vi "Read Tube Valves.vi"(0 "task in":refnum<k21>, 1 "Error In":errorcluster, 2 "Tube Inlet":bool, 3 "Mix Inlet":bool, 4 "Mix Outlet":bool, 5 "Tube Outlet":bool) -> (14 "task out":refnum<k21>, 15 "Error Out":errorcluster, 16 "Tube Inlet State":bool, 17 "Mix Inlet State":bool, 18 "Mix Outlet State":bool, 19 "Tube Outlet State":bool)   [LabVIEW 2018]
uses:
  <vilib>/DAQmx/write.llb/DAQmx Write (Digital 1D Bool 1Chan 1Samp).vi
  <vilib>/DAQmx/create/channels.llb/DAQmx Create Channel (DO-Digital Output).vi
  <vilib>/DAQmx/miscellaneous.llb/DAQmx Fill In Error Info.vi
panel:
  # "Valve Controls"
  # "TRUE:   valve open\nFALSE:  valve closed"
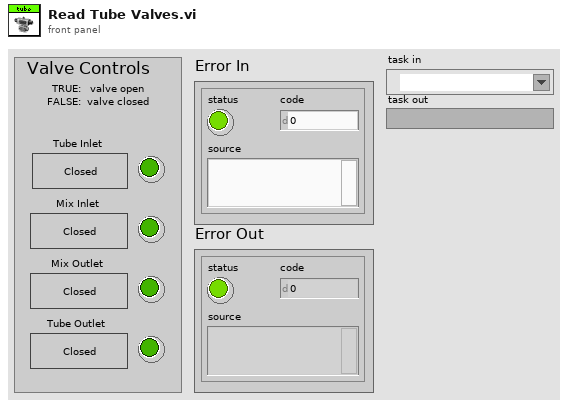
[diagram p1: front panel]
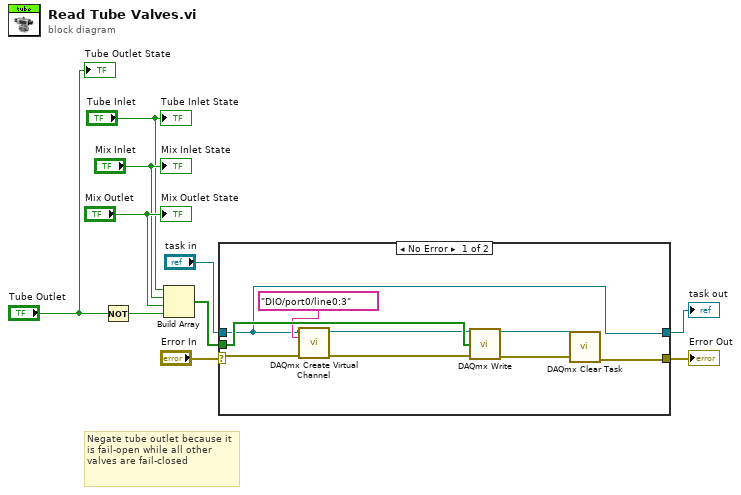
[diagram p0: block diagram]
diagram:
  # "Negate tube outlet because it is fail-open while all other valves are fail-closed"
  n1 = Not(x="Tube Outlet") -> (.not. x?=w8:bool)
  n2 = Build Array("Tube Inlet", "Mix Inlet", "Mix Outlet", w8) -> (w7:bool[])
  n3 = case shown="No Error" "Error In" {
    selector: "Error In" -> [w16 w21]
    tunnel: [w17 w21] -> w9
    tunnel: w7 -> [w19 _]
    tunnel: "task in" -> [w11 w20]
    tunnel: [w11 w20] -> w1
    frame No Error {
      n4 = call-poly <vilib>:"DAQmx Create Virtual Channel.vi"("task in"=w11, "lines"=tag "DIO/port0/line0:3", "error in"=w16) -> ("task out"=w13:refnum<k21>, "error out"=w15:errorcluster)  [unwired: 11 in]
      n5 = call-poly <vilib>:"DAQmx Write.vi"("task/channels in"=w13, "data"=w19, "error in"=w15) -> ("task out"=w12:refnum<k21>, "error out"=w14:errorcluster)  [unwired: 10 in, 1 out]
      n6 = call <vilib>:"DAQmx Clear Task.vi"("task in"=w12, "error in"=w14) -> ("error out"=w17:errorcluster)  [unwired: 13 in]
    }
    frame Error {
    }
  }
  "Error Out" <- w9
  "task out" <- w1
  "Tube Inlet State" <- "Tube Inlet"
  "Mix Inlet State" <- "Mix Inlet"
  "Mix Outlet State" <- "Mix Outlet"
  "Tube Outlet State" <- "Tube Outlet"
